vi "temperatur.vi"(8 "error in":errorcluster, 11 "Start":bool) -> (0 "error out":errorcluster, 2 "done":bool, 3 "Temperatur":dbl)   [LabVIEW 2013]
uses:
  <vilib>/DAQmx/create/channels.llb/DAQmx Create Channel (AI-Voltage-Basic).vi
  <vilib>/DAQmx/read.llb/DAQmx Read (Analog DBL 1Chan 1Samp).vi
panel:
  in  "U_gesamt":dbl=8.0 format="%#_13g"
  out "Numeric":dbl format="%#_13g"
  out "Ug - Ut":dbl
  out "widerstand":dbl
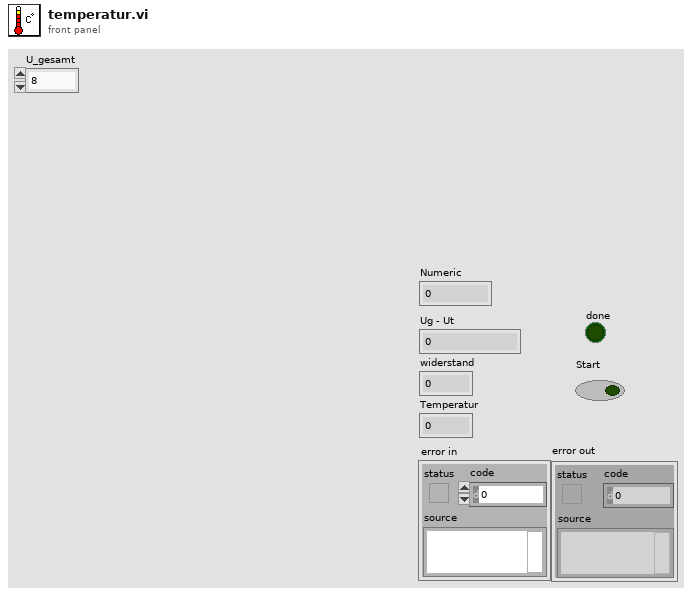
[diagram p1: front panel]
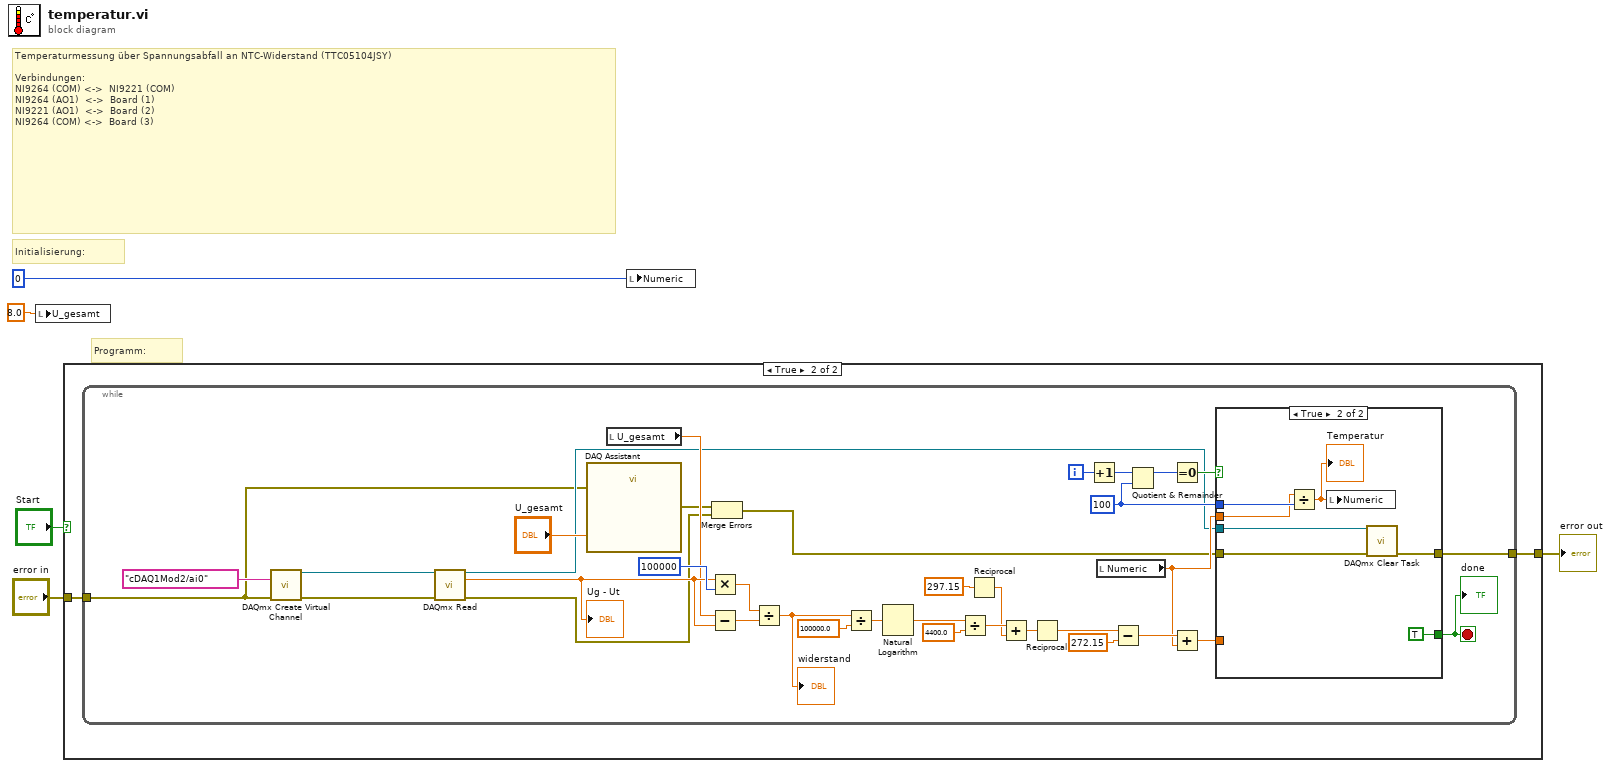
[diagram p0: block diagram]
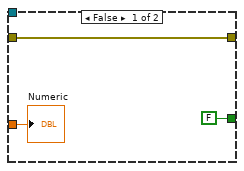
[diagram p3: hidden frame]
diagram:
  # "Programm:"
  # "Initialisierung:"
  # "Temperaturmessung über Spannungsabfall an NTC-Widerstand (TTC05104JSY)\n\nVerbindungen:  \nNI9264 (COM) <->  NI9221 (COM)\nNI9264 (AO1)  <->  Board (1)\nNI9221 (AO1)  <->  Board (2)\nNI9264 (COM) <->  Board (3)"
  n1 = local write "U_gesamt"(8.0 ("U_gesamt")) -> ()
  n2 = case shown="True" "Start" {
    tunnel: "error in" -> [w6 w8]
    tunnel: [w6 w7] -> w1
    frame False {
    }
    frame True {
      n3 = while {
        tunnel: w8 -> [w14]
        tunnel: [w10] -> w7
        i -> [w19]
        stop <- w16 stop-if-true
        w24 = 100 ("y")
        n4 = call-poly <vilib>:"DAQmx Create Virtual Channel.vi"("physical channels"=tag "cDAQ1Mod2/ai0", "error in"=w14) -> ("task out"=w22:refnum<k21>, "error out"=w13:errorcluster)  [unwired: 12 in]
        n5 = call-poly <vilib>:"DAQmx Read.vi"("task/channels in"=w22, "error in"=w13) -> ("task out"=w15:refnum<k21>, "data"=w23:dbl, "error out"=w11:errorcluster)  [unwired: 11 in]
        "Ug - Ut" <- w23
        n6 = call "DAQ Assistant"("data"="U_gesamt", "error in"=w14) -> ("error out"=w12:errorcluster)  [unwired: 16 in, 1 out]
        n7 = local read "U_gesamt"() -> (w20:dbl)
        n8 = Multiply(x=w23, y=100000) -> (x*y=w42:dbl)
        n9 = Subtract(x=w20, y=w23) -> (x-y=w41:dbl)
        n10 = Merge Errors(w12, w11) -> (w9:errorcluster)
        n11 = Divide(x=w42, y=w41) -> (x/y=w32:dbl)
        "widerstand" <- w32
        n12 = Divide(x=w32, y=100000.0) -> (x/y=w39:dbl)
        n13 = Natural Logarithm(1:w39) -> (0:w38:dbl)
        n14 = Divide(x=w38, y=4400.0) -> (x/y=w36:dbl)
        n15 = Reciprocal(x=297.15 ("y")) -> (1/x=w33:dbl)
        n16 = Add(x=w36, y=w33) -> (x+y=w35:dbl)
        n17 = Reciprocal(x=w35) -> (1/x=w31:dbl)
        n18 = Increment(x=w19) -> (x+1=w18:i32)
        n19 = local read "Numeric"() -> (w28:dbl)
        n20 = Subtract(x=w31, y=272.15) -> (x-y=w29:dbl)
        n21 = Quotient & Remainder(x=w18, y=w24) -> (x-y*floor(x/y)=w27:i32)  [unwired: 1 out]
        n22 = Equal To 0?(x=w27) -> (x = 0?=w26:bool)
        n23 = Add(x=w29, y=w28) -> (x+y=w25:dbl)
        n24 = case shown="True" w26 {
          tunnel: w24 -> [_ w53]
          tunnel: w28 -> [_ w52]
          tunnel: w25 -> [w46 _]
          tunnel: [FALSE TRUE] -> w16
          tunnel: w15 -> [_ w49]
          tunnel: [w44 w48] -> w10
          tunnel: w9 -> [w44 w47]
          frame False {
            "Numeric" <- w46
          }
          frame True {
            n25 = Divide(x=w52, y=w53) -> (x/y=w51:dbl)
            "Temperatur" <- w51
            n26 = local write "Numeric"(w51) -> ()
            n27 = call <vilib>:"DAQmx Clear Task.vi"("task in"=w49, "error in"=w47) -> ("error out"=w48:errorcluster)  [unwired: 13 in]
          }
        }
        "done" <- w16
      }
    }
  }
  "error out" <- w1
  n28 = local write "Numeric"(0) -> ()
